vi "Main.vi"() -> ()   [LabVIEW 2019]
uses:
  <vilib>/sound2/lvsound2.llb/Sampling Mode.ctl
  <vilib>/addons/_NISVFA/_Shared subVIs/Controls/svc_Engineering Units Text Ring.ctl
  <vilib>/addons/Sound and Vibration/svt_DAQmx/Configuration XControl/SVX NI-DAQmx AI Configuration XControl.xctl
  <vilib>/Utility/file.llb/Write Delimited Spreadsheet (string).vi
  <vilib>/Utility/file.llb/Read Delimited Spreadsheet (string).vi
  <vilib>/Utility/file.llb/Read Delimited Spreadsheet (DBL).vi
  GlobalVariable.vi
  <vilib>/express/express arith-compare/Formula/XNode/ExpressFormulaBlockNode.xnode
panel:
  in  "UI":T1(tab)
  in  "Path to output CSV file:":path
  in  "Path to input CSV file:":path
  in  "Weighting setting:":u16(ring)=1 items=["Linear", "A-weighting", "B-weighting", "C-weighting"]
  in  "Playback Device ID:":u32
  in  "channel info right":T3={"Sensitivity (mV/Pa):"=13.0, "Units:"=2, "dB reference:"=2e-05, "Pregain (dB):"=0.0} caption="Recording channel (right):" {"Pregain (dB):" format="%.2f"; "dB reference:" format="%^.1e"; "Units:" items=["custom..."=0, "V"=1, "A"=21, "C"=30, "pC"=31, "s"=32, "-"=29, "Pa"=2, "N"=20, "g"=3, "m/s^2"=4, "m/s"=5, "m"=6, "mm/s"=12, "mm"=13, "micron/s"=14, "micron"=15, "in/s^2"=7, "in/s"=8, "in"=9, "mil/s"=10, "mil"=11, "rad/s^2"=16, "rad/s"=17, "rad"=18, "deg/s^2"=26, "deg/s"=27, "deg"=28, "RPM"=22, "cycle/s^2"=23, "Hz"=24, "cycle"=25, "strain"=19]; "Sensitivity (mV/Pa):" format="%#_5f"}
  in  "channel info left":T3={"Sensitivity (mV/Pa):"=12.21, "Units:"=2, "dB reference:"=2e-05, "Pregain (dB):"=0.0} caption="Recording channel (left):" {"Pregain (dB):" format="%.2f"; "dB reference:" format="%^.1e"; "Units:" items=["custom..."=0, "V"=1, "A"=21, "C"=30, "pC"=31, "s"=32, "-"=29, "Pa"=2, "N"=20, "g"=3, "m/s^2"=4, "m/s"=5, "m"=6, "mm/s"=12, "mm"=13, "micron/s"=14, "micron"=15, "in/s^2"=7, "in/s"=8, "in"=9, "mil/s"=10, "mil"=11, "rad/s^2"=16, "rad/s"=17, "rad"=18, "deg/s^2"=26, "deg/s"=27, "deg"=28, "RPM"=22, "cycle/s^2"=23, "Hz"=24, "cycle"=25, "strain"=19]; "Sensitivity (mV/Pa):" format="%#_5f"}
  in  "Playback sample mode:":T4 items=["Finite Samples", "Continuous Samples"]
  in  "XControl Settings":refnum<k21>(xcontrol) caption="SVX NI-DAQmx AI Configuration XControl"
  out "Filepath:":path
  out "Number of tracks to calibrate:":i32
  out "Current gain (G):":dbl format="%#.4g"
  out "Current Leq (C):":dbl format="%#.4g"
  out "Lower limit (L):":dbl format="%#.4g"
  out "Upper limit (U):":dbl format="%#.4g"
  out "Flag (F):":dbl
  out "Final gain:":dbl format="%#.4g"
  out "Boundary search iteration (n):":i32
  out "Binary search iteration (n):":i32
  out "Total # of calls to MeasureLeq:":i32
  out "Progress (%):":dbl(slide) scale=0.0..100.0
  out "Adjusted initial guess:":dbl format="%#.4g"
  out "Final Leq:":dbl format="%#.4g"
  out "Tolerance (T):":dbl
  out "Desired Leq (D):":dbl
  out "Max. iterations for binary search (N):":i32
  out "Max. iterations for boundary search (N):":i32
  out "Multiplier (M):":i32
  out "Initial guess (G):":dbl
  out "Adjusting intial guess":bool
  out "Boundary search":bool
  out "Binary search":bool
  out "Sound Devices":cluster{"Device ID":u32, "Device Name":string}[](array[cluster])
  # "USER GUIDE\n\nThis LabVIEW Virtual Instrument (VI) helps you to automatically search for suitable gains to apply to audio tracks (mono or stereo) stored in a folder of your system to an Leq level (within a certain tolerance) that you can specify. The VI will output the values of these gains into a CSV file, which you can then apply to those audio tracks in order to calibrate them to the Leq level that you specified. Note that the original audio tracks are not modified in any way by the VI.\n\nThe VI searches for the suitable gains by firstly adjusting an initial guess based on an initial measurement. If the adjustment is not within the desired tolerance level, then a further boundary search, followed by a binary search, is used to refine the gain to the desired tolerance level. For more information on the calibration algorithm, please refer to our paper \"Automation of binaural headphone audio calibration on an artificial head\".\n\nThe steps to use this VI are as follows:\n                                                              \n1. Set overall parameters\n1) Under \"Path to input CSV file\", type in the path to the CSV file containing the filepaths for the tracks to calibrate, together with the input parameters for each track*.\n2) Under \"Path to output CSV file\", type in the path to the CSV file that you want to save the VI's output to. The VI will append to the rows of this CSV file if it already exists, and will the create the CSV file if it does not already exist**. \n\n2. Set Leq Measurement Parameters\n1) Under both \"Recording channel (left)\" and \"Recording channel (right)\", enter the corresponding sensitivity, units of measurement, value of the reference for dB calculation, and the pregain of the microphones corresponding to the left and right channels of the head and torso simulator, respectively.\n2) Under \"Playback Device ID\", enter the integer corresponding to the device ID of your playback device (which should normally be a pair of circumaural headphones or a soundcard). To check the device IDs of all playback/recording devices on your system, please refer to the tab \"X. Sound Device List\".\n3) Under \"Weighting setting\", select the weighting filter to be applied to the values recorded by the micrphones on the head and torso simulator.\n4) If necessary, the \"XControl Settings\" panel allows you to specify additional device settings according to your recording devices***. These include:\n     - \"NI-DAQmx Channel\" -- The names of the input channels corresponding to the left and right channels of the head and torso \n                             simulator. The left channel name should be above the right channel name in this column. E.g. if\n                             \"cDAQ1Mod1/ai1\" corresponds to the left channel and \"cDAQ1Mod1/ai0\" corresponds to the right\n                             channel, then the order in which the channels should appear in this column is \"cDAQ1Mod1/ai1\" on \n                             top, and \"cDAQ1Mod1/ai0\" at the bottom.\n     - \"Coupling\" -- The coupling mode for the microphones of the head and torso simulator.\n     - \"Excitation\" -- If your microphones (sensors) require excitation.\n\n3. Run VI (Ctrl+R) and Check Current Status\nThe \"3. Current Status\" tab will show the following items:\n    - \"Progress (%)\" -- The proportion of tracks for which an appropriate gain has been found to calibrate it to the desired \n                        Leq, expressed as a percentage. \n    - \"Number of tracks to calibrate\" -- Number of files to calibrate, as read by the VI from your input CSV file.\nInput parameters for current track: \n    - All input parameters for the current track as read from the input CSV file headers*.\nResults for current track:\n    - \"Adjusted initial guess\" -- The gain after the first adjustment to the initial guess (denoted as G' in our paper).\n    - \"Boundary search iteration (n)\" -- The current iteration of the boundary search, or 0 if boundary search has not started.\n    - \"Lower limit (L)\" -- The lower limit found by the boundary search, displayed after it has completed.\n    - \"Upper limit (U)\" -- The upper limit found by the boundary search, displayed after it has completed.\n    - \"Binary search iteration (n)\" -- The current iteration of the binary search, or 0 if the binary search has not started.\n    - \"Current gain (G)\" -- If the binary search has started, this will be the gain applied to the current audio track to obtain \n                            the Leq value in \"Current Leq (C)\". Otherwise, this will be 0.\n    - \"Current Leq (C)\" -- If the binary search has started, this will be the Leq value measured by the VI when the current \n                           audio track is played back at the gain value in \"Current gain (G)\". Otherise, this will be 0.\nFinal results for previous track:\n    - \"Final gain\" -- The gain that needs to be applied to the previous audio track to calibrate it to the value in \"Final Leq\".\n    - \"Final Leq\" -- The Leq value measured by the VI when the audio track is played back at the gain value in \"Final gain\".\n    - \"Total # of calls to MeasureLeq\" -- The number of times that MeasureLeq was called for the previous track.\n\nExpcept for \"Final results for previous results\", all the variables will be initialized to 0 at the end of each file and updated when callcalled.\n\nFootnotes\n*The input CSV file should contain a header row, followed by one row for every file that you want to calibrate. The header should contain the following columns in order:\n    - \"Filepath\" -- The path to the audio track to be calibrated (absolute path or relative path to the CSV file's directory). \n    - \"Desired Leq (D)\" -- The Leq that you wish to calibrate the current track to, in decibels.\n    - \"Tolernce (T)\" -- The tolerance of current track for the calibration, in decibels. T must be a positive real number.\n                        The VI will output a value of the gain that calibrates the track to an Leq in the range [D-T, D+T].\n    - \"Initial guess (G)\" -- Your initial guess for the gain. G must be a positive real number.\n    - \"Multiplier (M)\" -- The multiplier for the boundary search, which controls the coarseness of the boundary search.\n                          M must be a real number strictly greater than 1.\n                          In general, a larger value will allow the boundary search to converge more quickly,\n                          at the expense of a larger search space for the binary search.\n    - \"Max. iterations for boundary search (N)\" -- The maximum number of iterations allowed for the boundary search. The search\n                                                   is considered unsuccessful if the number of iterations exceeds this value.\n    - \"Max. iterations for binary search (N)\" -- The maximum number of iterations allowed for the binary search. The search\n                                                 is considered unsuccessful if the number of iterations exceeds this value.\n\n**The output CSV file will contain a header row, followed by one row for every non-header row in the input CSV file.\nThe header will contain the following columns in order:\n    - \"Filepath\" -- The path to the audio track to be calibrated.\n    - \"Gain\" -- A positive real number specifying the gain that needs to be applied to the audio track to calibrate it to the\n                value in \"Leq\" column. If the search is unsuccessful, the value will be -1.\n    - \"Leq\" -- The Leq value measured by the VI when the audio track is played back at the gain value in the \"Gain\" column.\n    - \"Calls to MeasureLeq\" -- The total number of times that the VI played back the audio track to obtain the value in the \n                               \"Gain\" column.\n    - \"Boundary search iterations\" -- The number of iterations taken for the boundary search for this audio track.\n    - \"Binary search iterations\" -- The number of iterations taken for the binary search for this audio track.\n    - \"Within range\" -- \"Y\" if the value in \"gain\" does not result in clipping of the audio track,\n                        and \"N\" if it results in clipping.\n    - \"Date\" -- System date when the VI accomplished searching for the audio track located at the path in \"Filepath\".\n    - \"Time\" -- System time when the VI accomplished searching for the audio track located at the path in \"Filepath\".\nIf many values in the \"Gain\" column are -1 (indicating many unsuccessful searches), try increasing the value of N, M, or T, in that order. If many values in the \"Within range\" column are \"N\", try increasing the physical gain of your system (e.g. turn up your volumn knob).\n\n***Note that values in the \"Master Settings\" panel will override those in the \"XControl Settings\" panel. If you encounter a \"memory is full\" error, try stopping the VI and running it again without changing any further settings. For further information, please refer to https://zone.ni.com/reference/en-XX/help/372416L-01/sndvibtk/daqmx_configuration/."
  # "1. Set overall parameters\n1) Under \"Path to input CSV file\", type in the path to the CSV file containing the filepaths for the tracks to calibrate, together with the input parameters for each track*.\n2) Under \"Path to output CSV file\", type in the path to the CSV file that you want to save the VI's output to. The VI will append to the rows of this CSV file if it already exists, and will the create the CSV file if it does not already exist**.\n\n*The input CSV file should contain a header row, followed by one row for every file that you want to calibrate. The header should contain the following columns in order:\n    - \"Filepath\" -- The path to the audio track to be calibrated (absolute path or relative path to the CSV file's directory). \n    - \"Desired Leq (D)\" -- The Leq that you wish to calibrate the current track to, in decibels.\n    - \"Tolernce (T)\" -- The tolerance of current track for the calibration, in decibels. T must be a positive real number.\n                        The VI will output a value of the gain that calibrates the track to an Leq in the range [D-T, D+T].\n    - \"Initial guess (G)\" -- Your initial guess for the gain. G must be a positive real number.\n    - \"Multiplier (M)\" -- The multiplier for the boundary search, which controls the coarseness of the boundary search.\n                          M must be a real number strictly greater than 1.\n                          In general, a larger value will allow the boundary search to converge more quickly,\n                          at the expense of a larger search space for the binary search.\n    - \"Max. iterations for boundary search (N)\" -- The maximum number of iterations allowed for the boundary search. The search\n                                                   is considered unsuccessful if the number of iterations exceeds this value.\n    - \"Max. iterations for binary search (N)\" -- The maximum number of iterations allowed for the binary search. The search\n                                                 is considered unsuccessful if the number of iterations exceeds this value.\n\n**The output CSV file will contain a header row, followed by one row for every non-header row in the input CSV file.\nThe header will contain the following columns in order:\n    - \"Filepath\" -- The path to the audio track to be calibrated.\n    - \"Gain\" -- A positive real number specifying the gain that needs to be applied to the audio track to calibrate it to the\n                value in \"Leq\" column. If the search is unsuccessful, the value will be -1.\n    - \"Leq\" -- The Leq value measured by the VI when the audio track is played back at the gain value in the \"Gain\" column.\n    - \"Calls to MeasureLeq\" -- The total number of times that the VI played back the audio track to obtain the value in the \n                               \"Gain\" column.\n    - \"Boundary search iterations\" -- The number of iterations taken for the boundary search for this audio track.\n    - \"Binary search iterations\" -- The number of iterations taken for the binary search for this audio track.\n    - \"Within range\" -- \"Y\" if the value in \"gain\" does not result in clipping of the audio track,\n                        and \"N\" if it results in clipping.\n    - \"Date\" -- System date when the VI accomplished searching for the audio track located at the path in \"Filepath\".\n    - \"Time\" -- System time when the VI accomplished searching for the audio track located at the path in \"Filepath\".\nIf many values in the \"Gain\" column are -1 (indicating many unsuccessful searches), try increasing the value of N, M, or T, in that order. If many values in the \"Within range\" column are \"N\", try increasing the physical gain of your system (e.g. turn up your volumn knob)."
  # "OVERALL PARAMETERS"
  # "2. Set Leq Measurement Parameters\n1) Under both \"Recording channel (left)\" and \"Recording channel (right)\", enter the corresponding sensitivity, units of measurement, value of the reference for dB calculation, and the pregain of the microphones corresponding to the left and right channels of the head and torso simulator, respectively.\n2) Under \"Playback Device ID\", enter the integer corresponding to the device ID of your playback device (which should normally be a pair of circumaural headphones or a soundcard). To check the device IDs of all playback/recording devices on your system, please refer to the tab \"X. Sound Device List\".\n3) Under \"Weighting setting\", select the weighting filter to be applied to the values recorded by the micrphones on the head and torso simulator.\n4) If necessary, the \"XControl Settings\" panel allows you to specify additional device settings according to your recording devices***. These include:\n     - \"NI-DAQmx Channel\" -- The names of the input channels corresponding to the left and right channels of the head and torso \n                             simulator. The left channel name should be above the right channel name in this column. E.g. if\n                             \"cDAQ1Mod1/ai1\" corresponds to the left channel and \"cDAQ1Mod1/ai0\" corresponds to the right\n                             channel, then the order in which the channels should appear in this column is \"cDAQ1Mod1/ai1\" on \n                             top, and \"cDAQ1Mod1/ai0\" at the bottom.\n     - \"Coupling\" -- The coupling mode for the microphones of the head and torso simulator.\n     - \"Excitation\" -- If your microphones (sensors) require excitation.\n\n***Note that values in the \"Master Settings\" panel will override those in the \"XControl Settings\" panel. If you encounter a \"memory is full\" error, try stopping the VI and running it again without changing any further settings. For further information, please refer to https://zone.ni.com/reference/en-XX/help/372416L-01/sndvibtk/daqmx_configuration/."
  # "LEQ MEASUREMENT SETTINGS"
  # "Master Settings"
  # "3. Run VI (Ctrl+R) and Check Current Status\nThe \"3. Current Status\" tab will show the following items:\n    - \"Progress (%)\" -- The proportion of tracks for which an appropriate gain has been found to calibrate it to the desired \n                        Leq, expressed as a percentage. \n    - \"Number of tracks to calibrate\" -- Number of files to calibrate, as read by the VI from your input CSV file.\nInput parameters for current track: \n    - All input parameters for the current track as read from the input CSV file headers*.\nResults for current track:\n    - \"Adjusted initial guess\" -- The gain after the first adjustment to the initial guess (denoted as G' in our paper).\n    - \"Boundary search iteration (n)\" -- The current iteration of the boundary search, or 0 if boundary search has not started.\n    - \"Lower limit (L)\" -- The lower limit found by the boundary search, displayed after it has completed.\n    - \"Upper limit (U)\" -- The upper limit found by the boundary search, displayed after it has completed.\n    - \"Binary search iteration (n)\" -- The current iteration of the binary search, or 0 if the binary search has not started.\n    - \"Current gain (G)\" -- If the binary search has started, this will be the gain applied to the current audio track to obtain \n                            the Leq value in \"Current Leq (C)\". Otherwise, this will be 0.\n    - \"Current Leq (C)\" -- If the binary search has started, this will be the Leq value measured by the VI when the current \n                           audio track is played back at the gain value in \"Current gain (G)\". Otherise, this will be 0.\nFinal results for previous track:\n    - \"Final gain\" -- The gain that needs to be applied to the previous audio track to calibrate it to the value in \"Final Leq\".\n    - \"Final Leq\" -- The Leq value measured by the VI when the audio track is played back at the gain value in \"Final gain\".\n    - \"Total # of calls to MeasureLeq\" -- The number of times that MeasureLeq was called for the previous track.\n\nExpcept for \"Final results for previous results\", all the variables will be initialized to 0 at the end of each file and updated when callcalled."
  # "CURRENT STATUS"
  # "Input parameters for current track:"
  # "Results for current track:"
  # "Final results for previous track:"
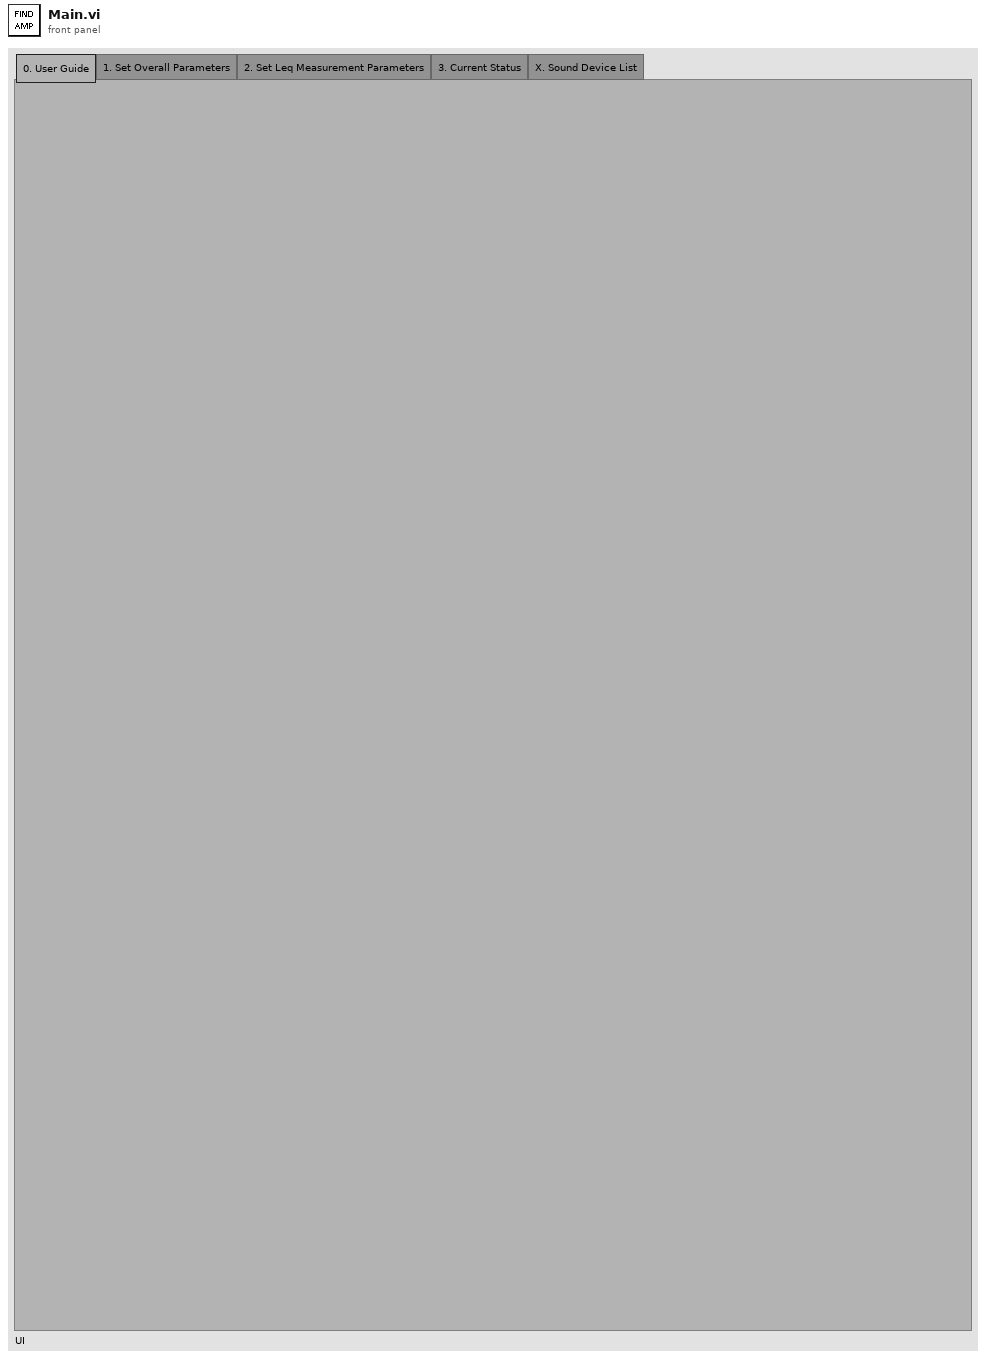
[diagram p1: front panel]
types:
  T1 = enum32{"0. User Guide", "1. Set Overall Parameters", "2. Set Leq Measurement Parameters", "3. Current Status", "X. Sound Device List"}
  T2 = typedef "svc_Engineering Units Text Ring.ctl" = u16
  T3 = cluster{"Sensitivity (mV/Pa):":dbl, "Units:":T2, "dB reference:":dbl, "Pregain (dB):":dbl}
  T4 = typedef "Sampling Mode.ctl" = i32
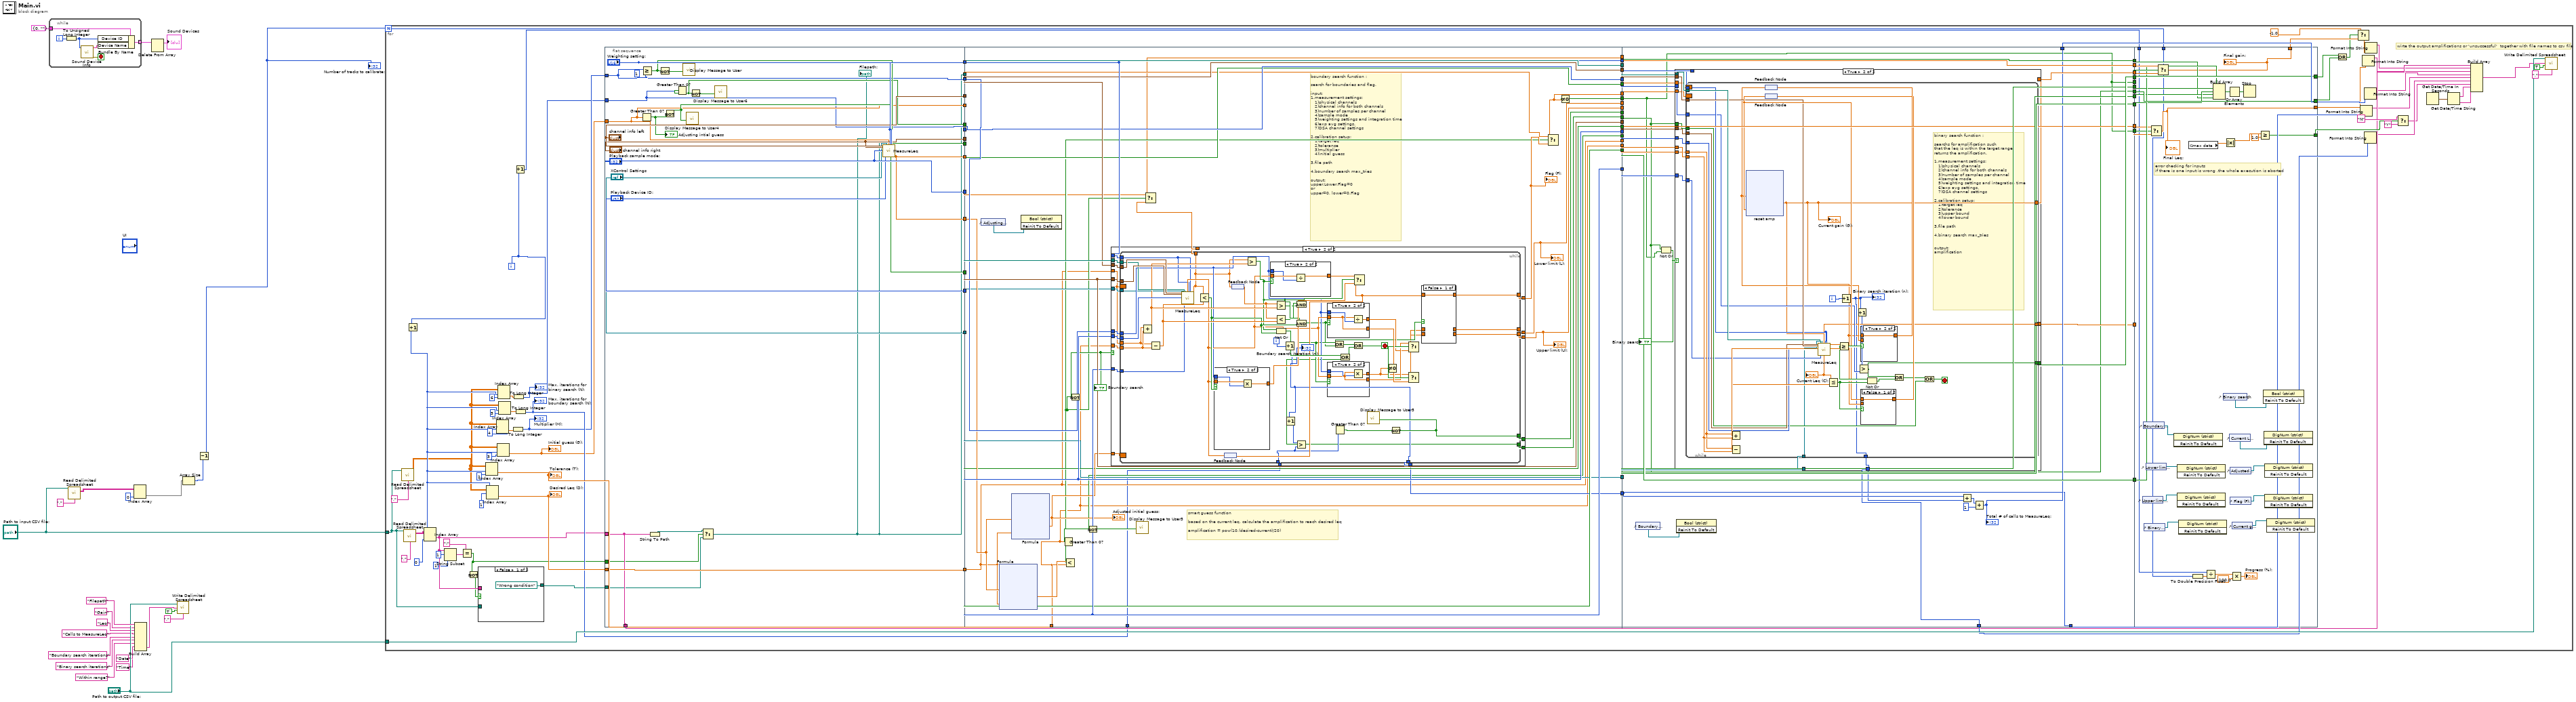
[diagram p0: block diagram]
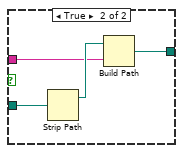
[diagram p2: hidden frame]
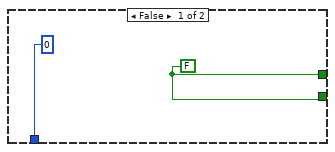
[diagram p3: hidden frame]
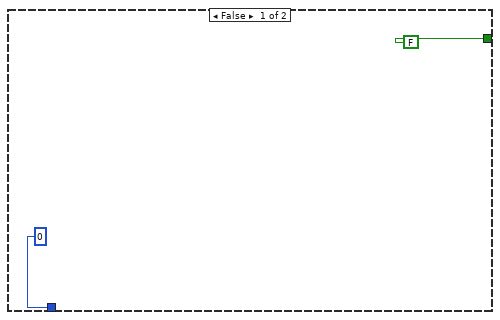
[diagram p9: hidden frame]
diagram:
  n1 = while {
    tunnel: cluster{"Device ID":u32, "Device Name":string} {"Device ID"=0, "Device Name"=""} ("入力クラスタ") -> [w27]
    tunnel: [w24] -> w22 mode=indexing
    i -> [w28]
    stop <- w29 stop-if-true
    n2 = To Unsigned Long Integer(number=w28) -> (unsigned 32bit integer=w26:u32)
    n3 = call <vilib>:"Sound Device Info.vi"("device"=w26) -> ("Device Name"=w25:string, "error out"=w29:errorcluster)  [unwired: 12 in, 1 out]
    n4 = Bundle By Name(cluster=w27, "Device ID"=w26, "Device Name"=w25) -> (w24:cluster{"Device ID":u32, "Device Name":string})
  }
  n5 = call-poly <vilib>:"Read Delimited Spreadsheet.vi"("file path (dialog if empty)"="Path to input CSV file:", "delimiter (\\t)"="," ("delimiter (\\t)")) -> ("all rows"=w5:string[][])  [unwired: 8 in, 5 out]
  n6 = Index Array(array=w5, index (col)=0 ("disabled index (col)")) -> (element=w3:string[])  [unwired: 1 in]
  n7 = Build Array("Filepath", "Gain" ("element"), "Leq" ("element"), "Calls to MeasureLeq" ("element"), "Boundary search iterations" ("element"), "Binary search iterations" ("element"), "Within range?" ("element"), "Date" ("element"), "Time" ("element")) -> (w17:string[])
  n8 = Delete From Array(array=w22) -> (array with subset deleted=→"Sound Devices":cluster{"Device ID":u32, "Device Name":string}[])  [unwired: 2 in, 1 out]
  n9 = call-poly <vilib>:"Write Delimited Spreadsheet.vi"("file path (dialog if empty)"="Path to output CSV file:", "1D data"=w17, "append to file? (new file:F)"=TRUE, "delimiter (\\t)"="," ("delimiter (\\t)")) -> ()  [unwired: 10 in, 2 out]
  n10 = Array Size(array=w3) -> (size(s)=w2:i32)
  n11 = Decrement(x=w2) -> (x-1=w1:i32)
  "Number of tracks to calibrate:" <- w1
  n12 = for {
    N: w1 -> [w39]
    tunnel: "Path to output CSV file:" -> [w138]
    tunnel: "Path to input CSV file:" -> [w38]
    i -> [w61]
    # "wirte the output amplifications or 'unsuccessful'  together with file names to csv file"
    n13 = call-poly <vilib>:"Read Delimited Spreadsheet.vi"("file path (dialog if empty)"=w38, "delimiter (\\t)"="," ("delimiter (\\t)")) -> ("all rows"=w43:dbl[][])  [unwired: 8 in, 5 out]
    n14 = call-poly <vilib>:"Read Delimited Spreadsheet.vi"("file path (dialog if empty)"=w38, "delimiter (\\t)"="," ("delimiter (\\t)")) -> ("all rows"=w59:string[][])  [unwired: 8 in, 5 out]
    n15 = Increment(x=w61) -> (x+1=w44:i32)
    n16 = Index Array(array=w59, index (row)=w44, index (col)=0 ("disabled index (col)")) -> (element=w37:string)
    n17 = String Subset(string=w37, offset (0)=1, length (rest)=1 ("length (rest)")) -> (substring=w34:string)
    n18 = Equal?(x=":", y=w34) -> (x = y?=w31:bool)
    n19 = Not(x=w31) -> (.not. x?=w30:bool)
    n20 = case shown="False" w30 {
      tunnel: w38 -> [_ w145]
      tunnel: w37 -> [_ w143]
      tunnel: [path "Wrong condition" ("appended path") w142] -> w32
      frame False {
      }
      frame True {
        n21 = Strip Path(path=w145) -> (stripped path=w144:path)  [unwired: 1 out]
        n22 = Build Path(base path=w144, name or relative path=w143) -> (appended path=w142:path)
      }
    }
    n23 = Index Array(array=w43, index (row)=w44, index (col)=2 ("disabled index (col)")) -> (element=w55:dbl)
    "Tolerance (T):" <- w55
    n24 = Index Array(array=w43, index (row)=w44, index (col)=1 ("disabled index (col)")) -> (element=w56:dbl)
    "Desired Leq (D):" <- w56
    n25 = Index Array(array=w43, index (row)=w44, index (col)=4) -> (element=w51:dbl)
    n26 = Index Array(array=w43, index (row)=w44, index (col)=3) -> (element=w47:dbl)
    "Initial guess (G):" <- w47
    n27 = Index Array(array=w43, index (row)=w44, index (col)=6) -> (element=w42:dbl)
    n28 = Index Array(array=w43, index (row)=w44, index (col)=5 ("disabled index (col)")) -> (element=w49:dbl)
    n29 = To Long Integer(number=w51) -> (32bit integer=w46:i32)
    "Multiplier (M):" <- w46
    n30 = To Long Integer(number=w42) -> (32bit integer=w41:i32)
    "Max. iterations for binary search (N):" <- w41
    n31 = Increment(x=w61) -> (x+1=w40:i32)
    n32 = To Long Integer(number=w49) -> (32bit integer=w48:i32)
    "Max. iterations for boundary search (N):" <- w48
    n33 = flat-sequence {
      tunnel: [w150] -> w140
      tunnel: [w154] -> w85
      tunnel: ["Weighting setting:"] -> w106
      tunnel: ["channel info left"] -> w105
      tunnel: ["channel info right"] -> w104
      tunnel: ["Playback sample mode:"] -> w103
      tunnel: [w152] -> w102
      tunnel: ["Playback Device ID:"] -> w101
      tunnel: [w156] -> w100
      tunnel: [w157] -> w99
      tunnel: [w161] -> w98
      tunnel: [w151] -> w97
      tunnel: [w158] -> w96
      tunnel: [w153] -> w95
      tunnel: ["XControl Settings"] -> w87
      tunnel: [w156] -> w64
      tunnel: w37 -> [w154]
      tunnel: [w155] -> w57
      tunnel: w56 -> [w155]
      tunnel: w47 -> [w153]
      tunnel: w46 -> [w152]
      tunnel: w41 -> [w151]
      tunnel: w32 -> [w148]
      tunnel: w31 -> [w147]
      tunnel: w140 -> [w203]
      tunnel: [w182] -> w136
      tunnel: [w181] -> w135
      tunnel: [w203] -> w134
      tunnel: [w198] -> w133
      tunnel: [w197] -> w132
      tunnel: [w196] -> w131
      tunnel: [w202] -> w130
      tunnel: [w185] -> w127
      tunnel: [w201] -> w122
      tunnel: [w171] -> w121
      tunnel: [w172] -> w120
      tunnel: [w194] -> w119
      tunnel: [w192] -> w118
      tunnel: [w177] -> w117
      tunnel: [w189] -> w116
      tunnel: [w200] -> w115
      tunnel: [w199] -> w109
      tunnel: [w188] -> w108
      tunnel: [w187] -> w107
      tunnel: w106 -> [w199]
      tunnel: w105 -> [w198]
      tunnel: w104 -> [w197]
      tunnel: w103 -> [w196]
      tunnel: w102 -> [w195]
      tunnel: w101 -> [w194]
      tunnel: w100 -> [w191]
      tunnel: w99 -> [w192]
      tunnel: w98 -> [w189]
      tunnel: w97 -> [w188]
      tunnel: w96 -> [w187]
      tunnel: w95 -> [w186]
      tunnel: [w184] -> w94
      tunnel: w87 -> [w179]
      tunnel: [w179] -> w86
      tunnel: [w173] -> w81
      tunnel: w64 -> [w175]
      tunnel: w57 -> [w172]
      tunnel: w55 -> [w171]
      tunnel: w48 -> [w170]
      tunnel: w136 -> [w331]
      tunnel: w135 -> [w330]
      tunnel: w134 -> [w337]
      tunnel: w133 -> [w336]
      tunnel: w132 -> [w335]
      tunnel: w131 -> [w334]
      tunnel: w130 -> [w308]
      tunnel: [w308] -> w129
      tunnel: [w333] -> w128
      tunnel: w127 -> [w333]
      tunnel: [w332] -> w126
      tunnel: [w329] -> w125
      tunnel: [w309] -> w123
      tunnel: w122 -> [w309]
      tunnel: w121 -> [w328]
      tunnel: w120 -> [w327]
      tunnel: w119 -> [w326]
      tunnel: w118 -> [w325]
      tunnel: w117 -> [w324]
      tunnel: w116 -> [w323]
      tunnel: w115 -> [w322]
      tunnel: [w325] -> w114
      tunnel: [w324] -> w113
      tunnel: [w323] -> w112
      tunnel: [w322] -> w111
      tunnel: [w319] -> w110
      tunnel: w109 -> [w321]
      tunnel: w108 -> [w320]
      tunnel: w107 -> [w319]
      tunnel: w94 -> [w312]
      tunnel: [w316] -> w93
      tunnel: [w312] -> w91
      tunnel: [w311] -> w92
      tunnel: w86 -> [w315]
      tunnel: [w308] -> w83
      tunnel: [w314] -> w82
      tunnel: w81 -> [w314]
      tunnel: [w313] -> w80
      tunnel: w129 -> [w434]
      tunnel: w128 -> [w433]
      tunnel: w126 -> [w432]
      tunnel: [w419] -> w71
      tunnel: [w431] -> w124
      tunnel: w125 -> [w431]
      tunnel: [w430] -> w73
      tunnel: w123 -> [w430]
      tunnel: w114 -> [w429]
      tunnel: w113 -> [w428]
      tunnel: w112 -> [w427]
      tunnel: w111 -> [w426]
      tunnel: w110 -> [w425]
      tunnel: [w420] -> w89
      tunnel: w83 -> [w417]
      tunnel: w82 -> [w416]
      tunnel: w80 -> [w415]
      tunnel: [w414] -> w79
      tunnel: w40 -> [w409]
      tunnel: w39 -> [w408]
      frame #0 {
        n34 = Greater Than 0?(x=w153) -> (x > 0?=w146:bool)
        "Adjusting intial guess" <- w146
        n35 = Greater Or Equal?(x=w152, y=1) -> (x >= y?=w163:bool)
        n36 = String To Path(string=w154) -> (path=w149:path)
        n37 = Not(x=w163) -> (.not. x?=w161:bool)
        n38 = Not(x=w146) -> (.not. x?=w157:bool)
        n39 = Greater Than 0?(x=w151) -> (x > 0?=w159:bool)
        n40 = call "Display Message to User"("Enable"=w161) -> ()  [unwired: 9 in, 2 out]
        n41 = call "Display Message to User4"("Enable"=w157) -> ()  [unwired: 9 in, 2 out]
        n42 = Not(x=w159) -> (.not. x?=w158:bool)
        n43 = Select(t=w149, s=w147, f=w148) -> (s? t:f=w150:path)
        "Filepath:" <- w150
        n44 = call "Display Message to User6"("Enable"=w158) -> ()  [unwired: 9 in, 2 out]
        n45 = call "MeasureLeq.vi"("channel info left(necessary)"="channel info left", "channel info right (necessary)"="channel info right", "sample mode"="Playback sample mode:", "path"=w150, "device ID"="Playback Device ID:", "task"="XControl Settings", "Amplification"=w153, "weighting 2"="Weighting setting:", "weighting 3"="Weighting setting:") -> ("Leq sound level [dB EU] 4"=w156:dbl)  [unwired: 16 in, 2 out]
      }
      frame #1 {
        # "smart guess function\n\nbased on the current leq, calculate the amplification to reach desired leq\n\namplification = pow(10,(desired-current)/20)"
        # "boundary search function :\n\nsearch for boundaries and flag.\n\ninput: \n1.measurement settings:\n   1)physical channels\n   2)channel info for both channels\n   3)number of samples per channel\n   4)sample mode\n   5)weighting settings and integration time\n   6)exp avg settings.\n   7)DSA channel settings\n \n2.calibration setup:\n   1)target leq\n   2)tolerance\n   3)multiplier\n   4)initial guess\n\n3.file path\n\n4.boundary search max_tries \n\noutput:\nupper,Lower,Flag=0\nor\nupper=0, lower=0,Flag"
        n46 = control-ref of="Adjusting intial guess"() -> (w169:refnum<vi>)
        n47 = xnode "Formula"("current"=w191, "desired"=w172) -> ("Result"=w190:dbl)  [unwired: 1 in, 1 out]
        n48 = xnode ("Formula")("current"=w191, "desired"=w172) -> ("Result"=w193:dbl)  [unwired: 1 in, 1 out]
        "Adjusted initial guess:" <- w193
        n49 = invoke class="Bool (strict)" method="Reinit To Default"(reference=w169) -> ()  [unwired: 2 in, 3 out]
        n50 = Greater Than 0?(x=w171) -> (x > 0?=w178:bool)
        n51 = Less?(x=w190, y=w171) -> (x < y?=w176:bool)
        n52 = Not(x=w176) -> (.not. x?=w183:bool)
        "Boundary search" <- w183
        n53 = Not(x=w178) -> (.not. x?=w177:bool)
        n54 = case shown="True" w183 {
          tunnel: [_ w224] -> w182
          tunnel: [_ w223] -> w181
          tunnel: w203 -> [_ w222]
          tunnel: [w205 w221] -> w201
          tunnel: [w205 w220] -> w200
          tunnel: w199 -> [_ w219]
          tunnel: w198 -> [_ w218]
          tunnel: w197 -> [_ w217]
          tunnel: w196 -> [_ w216]
          tunnel: w195 -> [_ w215]
          tunnel: w194 -> [_ w214]
          tunnel: w193 -> [_ w213]
          tunnel: w172 -> [_ w206]
          tunnel: w171 -> [_ w212]
          tunnel: [_ w211] -> w180
          tunnel: [0 w210] -> w184
          tunnel: w179 -> [_ w209]
          tunnel: [_ w208] -> w174
          tunnel: w170 -> [_ w207]
          frame False {
            w205 = FALSE
          }
          frame True {
            n55 = while {
              tunnel: [w268] -> w224
              tunnel: [w267] -> w223
              tunnel: [w265] -> w211
              tunnel: w206 -> [w261]
              tunnel: w212 -> [w262]
              tunnel: w222 -> [w257]
              tunnel: w216 -> [w258]
              tunnel: w215 -> [w248]
              tunnel: w218 -> [w260]
              tunnel: w217 -> [w259]
              tunnel: [w225] -> w221
              tunnel: w214 -> [w236]
              border: w206 -> [_]
              tunnel: [w230] -> w220
              tunnel: w219 -> [w234]
              border: w213 -> [_]
              tunnel: [w227] -> w210
              tunnel: w209 -> [w232]
              tunnel: [w231] -> w208
              tunnel: w207 -> [w229]
              i -> [w228]
              stop <- w233 stop-if-true
              n56 = Add(x=w261, y=w262) -> (x+y=w256:dbl)
              n57 = Subtract(x=w261, y=w262) -> (x-y=w254:dbl)
              n58 = feedback #1() -> (w249:dbl)
              n59 = call "MeasureLeq.vi"("channel info left(necessary)"=w260, "channel info right (necessary)"=w259, "sample mode"=w258, "path"=w257, "device ID"=w236, "task"=w232, "Amplification"=w249, "weighting 2"=w234, "weighting 3"=w234) -> ("Leq sound level [dB EU] 4"=w231:dbl)  [unwired: 16 in, 2 out]
              n60 = Less?(x=w231, y=w254) -> (x < y?=w252:bool)
              n61 = case shown="True" w252 {
                tunnel: w249 -> [w279 w282]
                tunnel: [w279 w281] -> w264
                tunnel: w248 -> [_ w280]
                frame False {
                }
                frame True {
                  n62 = Multiply(x=w282, y=w280) -> (x*y=w281:dbl)
                }
              }
              n63 = feedback-in #2(w231) -> ()
              n64 = feedback #2() -> (w255:dbl)
              n65 = Greater?(x=w231, y=w256) -> (0:w250:bool)
              n66 = case shown="True" w250 {
                tunnel: w249 -> [w283 w286]
                tunnel: [w283 w285] -> w263
                tunnel: w248 -> [_ w284]
                frame False {
                }
                frame True {
                  n67 = Divide(x=w286, y=w284) -> (x/y=w285:dbl)
                }
              }
              n68 = Greater?(x=w255, y=w256) -> (0:w253:bool)
              n69 = Less?(x=w255, y=w254) -> (x < y?=w251:bool)
              n70 = Not Or(1:w252, 2:w250) -> (0:w269:bool)
              n71 = Increment(x=w228) -> (x+1=w227:i32)
              "Boundary search iteration (n):" <- w227
              n72 = Increment(x=w227) -> (x+1=w226:i32)
              n73 = Greater?(x=w226, y=w229) -> (0:w225:bool)
              n74 = And(x=w251, y=w250) -> (x .and. y?=w246:bool)
              n75 = And(x=w253, y=w252) -> (x .and. y?=w247:bool)
              n76 = case shown="True" w246 {
                tunnel: w249 -> [_ w270]
                tunnel: w248 -> [_ w272]
                tunnel: [_ w271] -> w241
                tunnel: [_ w270] -> w244
                frame False {
                }
                frame True {
                  n77 = Divide(x=w270, y=w272) -> (x/y=w271:dbl)
                }
              }
              n78 = case shown="True" w247 {
                tunnel: [_ w274] -> w242
                tunnel: w249 -> [_ w274]
                tunnel: w248 -> [_ w275]
                tunnel: [_ w273] -> w237
                frame False {
                }
                frame True {
                  n79 = Multiply(x=w274, y=w275) -> (x*y=w273:dbl)
                }
              }
              n80 = Or(x=w247, y=w246) -> (x .or. y?=w240:bool)
              n81 = Greater Than 0?(x=w229) -> (x > 0?=w235:bool)
              n82 = Or(x=w269, y=w225) -> (x .or. y?=w245:bool)
              n83 = Or(x=w240, y=w245) -> (x .or. y?=w233:bool)
              n84 = Select(t=w263, s=w250, f=w264) -> (s? t:f=w266:dbl)
              n85 = feedback-in #1(w266) -> ()
              n86 = Not Equal To 0?(x=w237) -> (x != 0?=w243:bool)
              n87 = Not(x=w235) -> (.not. x?=w230:bool)
              n88 = call "Display Message to User5"("Enable"=w230) -> ()  [unwired: 9 in, 2 out]
              n89 = Select(t=w242, s=w243, f=w241) -> (s? t:f=w238:dbl)
              n90 = Select(t=w237, s=w243, f=w244) -> (s? t:f=w239:dbl)
              n91 = case shown="False" w240 {
                tunnel: w238 -> [_ w278]
                tunnel: [_ w278] -> w268
                tunnel: [_ w277] -> w267
                tunnel: w239 -> [_ w277]
                tunnel: w266 -> [w276 _]
                tunnel: [w276 _] -> w265
                frame False {
                }
                frame True {
                }
              }
            }
          }
        }
        "Lower limit (L):" <- w182
        "Upper limit (U):" <- w181
        "Flag (F):" <- w180
        n92 = call "Display Message to User3"("Enable"=w177) -> ()  [unwired: 9 in, 2 out]
        n93 = Select(t=w175, s=w176, f=w174) -> (s? t:f=w173:dbl)
        n94 = Select(t=w186, s=w176, f=w180) -> (s? t:f=w185:dbl)
        n95 = Not Equal To 0?(x=w185) -> (x != 0?=w202:bool)
      }
      frame #2 {
        n96 = control-ref of="Boundary search"() -> (w307:refnum<vi>)
        n97 = Not Or(1:w308, 2:w309) -> (0:w310:bool)
        "Binary search" <- w310
        n98 = case shown="True" w310 {
          tunnel: w337 -> [_ w356]
          tunnel: w336 -> [_ w355]
          tunnel: w335 -> [_ w354]
          tunnel: w334 -> [_ w353]
          tunnel: [_ w352] -> w332
          tunnel: w331 -> [_ w351]
          tunnel: w330 -> [_ w350]
          tunnel: [FALSE w349] -> w329
          tunnel: w328 -> [_ w348]
          tunnel: w327 -> [_ w347]
          tunnel: w309 -> [_ w346]
          tunnel: w326 -> [_ w345]
          tunnel: w321 -> [_ w344]
          tunnel: w320 -> [_ w343]
          tunnel: [0 w342] -> w311
          tunnel: w315 -> [_ w341]
          tunnel: [_ w340] -> w313
          frame False {
          }
          frame True {
            n99 = while {
              tunnel: w356 -> [w376]
              tunnel: w355 -> [w375]
              tunnel: w354 -> [w374]
              tunnel: w353 -> [w373]
              tunnel: [w361] -> w352
              border: w351 -> [_]
              border: w350 -> [_]
              tunnel: [w372] -> w349
              tunnel: w348 -> [w371]
              tunnel: w347 -> [w370]
              tunnel: w346 -> [w369]
              tunnel: w345 -> [w366]
              tunnel: w344 -> [w365]
              tunnel: w343 -> [w364]
              tunnel: [w357] -> w342
              tunnel: w341 -> [w360]
              tunnel: [w359] -> w340
              i -> [w362]
              stop <- w368 stop-if-true
              # "binary search function :\n\nsearchs for amplification such \nthat the leq is within the target range.\nreturns the amplification. \n\n1.measurement settings:\n   1)physical channels\n   2)channel info for both channels\n   3)number of samples per channel\n   4)sample mode\n   5)weighting settings and integration time\n   6)exp avg settings.\n   7)DSA channel settings\n \n2.calibration setup:\n   1)target leq\n   2)tolerance\n   3)upper bound\n   4)lower bound\n\n3.file path\n\n4.binary search max_tries \n\n\noutput:\namplification"
              n100 = Add(x=w370, y=w371) -> (x+y=w384:dbl)
              n101 = Subtract(x=w370, y=w371) -> (x-y=w383:dbl)
              n102 = feedback #3() -> (w367:dbl)
              n103 = feedback #4() -> (w377:dbl)
              n104 = xnode ("reset amp")("upper"=w367, "lower"=w377) -> ("Result"=w361:dbl)  [unwired: 1 in, 1 out]
              "Current gain (G):" <- w361
              n105 = call "MeasureLeq.vi"("channel info left(necessary)"=w374, "channel info right (necessary)"=w375, "sample mode"=w373, "path"=w376, "device ID"=w366, "task"=w360, "Amplification"=w361, "weighting 2"=w365, "weighting 3"=w365) -> ("Leq sound level [dB EU] 4"=w359:dbl)  [unwired: 16 in, 2 out]
              "Current Leq (C):" <- w359
              n106 = Less Or Equal?(x=w359, y=w383) -> (x <= y?=w379:bool)
              n107 = Greater Or Equal?(x=w359, y=w384) -> (x >= y?=w380:bool)
              n108 = Increment(x=w362) -> (x+1=w357:i32)
              "Binary search iteration (n):" <- w357
              n109 = Increment(x=w357) -> (x+1=w358:i32)
              n110 = Greater?(x=w358, y=w364) -> (0:w372:bool)
              n111 = case shown="True" w380 {
                tunnel: w361 -> [_ w388]
                tunnel: [w387 w388] -> w382
                tunnel: w367 -> [w387 _]
                frame False {
                }
                frame True {
                }
              }
              n112 = feedback-in #3(w382) -> ()
              n113 = case shown="False" w379 {
                tunnel: w361 -> [_ w386]
                tunnel: [w385 w386] -> w381
                tunnel: w377 -> [w385 _]
                frame False {
                }
                frame True {
                }
              }
              n114 = feedback-in #4(w381) -> ()
              n115 = Not Or(1:w379, 2:w380) -> (0:w378:bool)
              n116 = Or(x=w372, y=w378) -> (x .or. y?=w363:bool)
              n117 = Or(x=w363, y=w369) -> (x .or. y?=w368:bool)
            }
          }
        }
        n118 = invoke class="Bool (strict)" method="Reinit To Default"(reference=w307) -> ()  [unwired: 2 in, 3 out]
        n119 = Add(x=w312, y=w311) -> (x+y=w318:i32)
        n120 = Add(x=w318, y=1) -> (x+y=w316:i32)
        "Total # of calls to MeasureLeq:" <- w316
      }
      frame #3 {
        # "error checking for inputs\nif there is one input is wrong ,the whole execution is aborted"
        n121 = control-ref of="Upper limit (U):"() -> (w402:refnum<vi>)
        n122 = control-ref of="Boundary search iteration (n):"() -> (w400:refnum<vi>)
        n123 = control-ref of="Binary search iteration (n):"() -> (w403:refnum<vi>)
        n124 = control-ref of="Lower limit (L):"() -> (w401:refnum<vi>)
        n125 = Select(t=w416, s=w417, f=w415) -> (s? t:f=w414:dbl)
        "Final Leq:" <- w414
        n126 = Select(t=w433, s=w434, f=w432) -> (s? t:f=w419:dbl)
        "Final gain:" <- w419
        n127 = invoke class="DigNum (strict)" method="Reinit To Default"(reference=w400) -> ()  [unwired: 2 in, 3 out]
        n128 = invoke class="DigNum (strict)" method="Reinit To Default"(reference=w402) -> ()  [unwired: 2 in, 3 out]
        n129 = invoke class="DigNum (strict)" method="Reinit To Default"(reference=w401) -> ()  [unwired: 2 in, 3 out]
        n130 = invoke class="DigNum (strict)" method="Reinit To Default"(reference=w403) -> ()  [unwired: 2 in, 3 out]
        n131 = global read "GlobalVariable.vi" "max data"() -> (w422:dbl)
        n132 = To Double Precision Float(number=w408) -> (double precision float=w411:dbl)
        n133 = Divide(x=w409, y=w411) -> (x/y=w412:dbl)
        n134 = Build Array(w429, w428, w427, w426, w425) -> (w424:bool[])
        n135 = control-ref of="Binary search"() -> (w399:refnum<vi>)
        n136 = Absolute Value(x=w422) -> (abs(x)=w418:dbl)
        n137 = Or Array Elements(Boolean array=w424) -> (logical OR=w423:bool)
        n138 = control-ref of="Current Leq (C):"() -> (w405:refnum<vi>)
        n139 = control-ref of="Adjusted initial guess:"() -> (w406:refnum<vi>)
        n140 = control-ref of="Flag (F):"() -> (w407:refnum<vi>)
        n141 = Multiply(x=w412, y=100.0) -> (x*y=→"Progress (%):":dbl)
        n142 = control-ref of="Current gain (G):"() -> (w404:refnum<vi>)
        n143 = Stop(stop? (T)=w423) -> ()
        n144 = Greater Or Equal?(x=w418, y=1.0) -> (x >= y?=w420:bool)
        n145 = invoke class="Bool (strict)" method="Reinit To Default"(reference=w399) -> ()  [unwired: 2 in, 3 out]
        n146 = invoke class="DigNum (strict)" method="Reinit To Default"(reference=w405) -> ()  [unwired: 2 in, 3 out]
        n147 = invoke class="DigNum (strict)" method="Reinit To Default"(reference=w406) -> ()  [unwired: 2 in, 3 out]
        n148 = invoke class="DigNum (strict)" method="Reinit To Default"(reference=w407) -> ()  [unwired: 2 in, 3 out]
        n149 = invoke class="DigNum (strict)" method="Reinit To Default"(reference=w404) -> ()  [unwired: 2 in, 3 out]
      }
    }
    n150 = Or(x=w124, y=w73) -> (x .or. y?=w69:bool)
    n151 = Select(t=-1.0, s=w69, f=w71) -> (s? t:f=w70:dbl)
    n152 = Format Into String(w91) -> (resulting string=w76:string)  [unwired: 3 in, 1 out]
    n153 = Format Into String(w79) -> (resulting string=w78:string)  [unwired: 3 in, 1 out]
    n154 = Format Into String(w92) -> (resulting string=w75:string)  [unwired: 3 in, 1 out]
    n155 = Format Into String(w93) -> (resulting string=w77:string)  [unwired: 3 in, 1 out]
    n156 = Format Into String(w70) -> (resulting string=w84:string)  [unwired: 3 in, 1 out]
    n157 = Select(t="N", s=w89, f="Y") -> (s? t:f=w74:string)
    n158 = Get Date/Time In Seconds() -> (seconds since 1Jan1904=w67:timestamp)
    n159 = Get Date/Time String(seconds (now)=w67) -> (date string=w66:string, time string=w65:string)  [unwired: 2 in]
    n160 = Build Array(w85, w84, w78, w77, w76, w75, w74, w66, w65) -> (w68:string[])
    n161 = call-poly <vilib>:"Write Delimited Spreadsheet.vi"("file path (dialog if empty)"=w138, "1D data"=w68, "append to file? (new file:F)"=TRUE, "delimiter (\\t)"="," ("delimiter (\\t)")) -> ()  [unwired: 10 in, 2 out]
  }
